vi "Programacion paralela.vi"() -> ()   [LabVIEW 2020]
panel:
  out "Thermometer 6":u16(slide) scale=0.0..100.0
  out "Thermometer 5":u16(slide) scale=0.0..100.0
  out "Thermometer 4":u16(slide) scale=0.0..100.0
  out "Thermometer 3":u16(slide) scale=0.0..100.0
  out "Thermometer 2":u16(slide) scale=0.0..100.0
  out "Thermometer":u16(slide) scale=0.0..100.0
  # "´Programacion PARALELA"
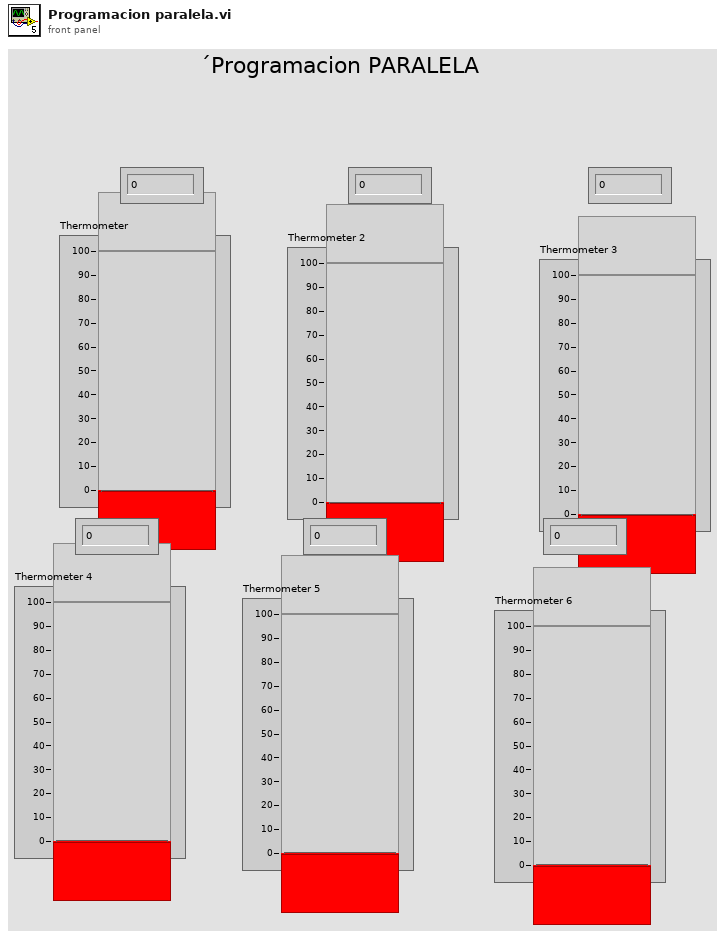
[diagram p1: front panel]
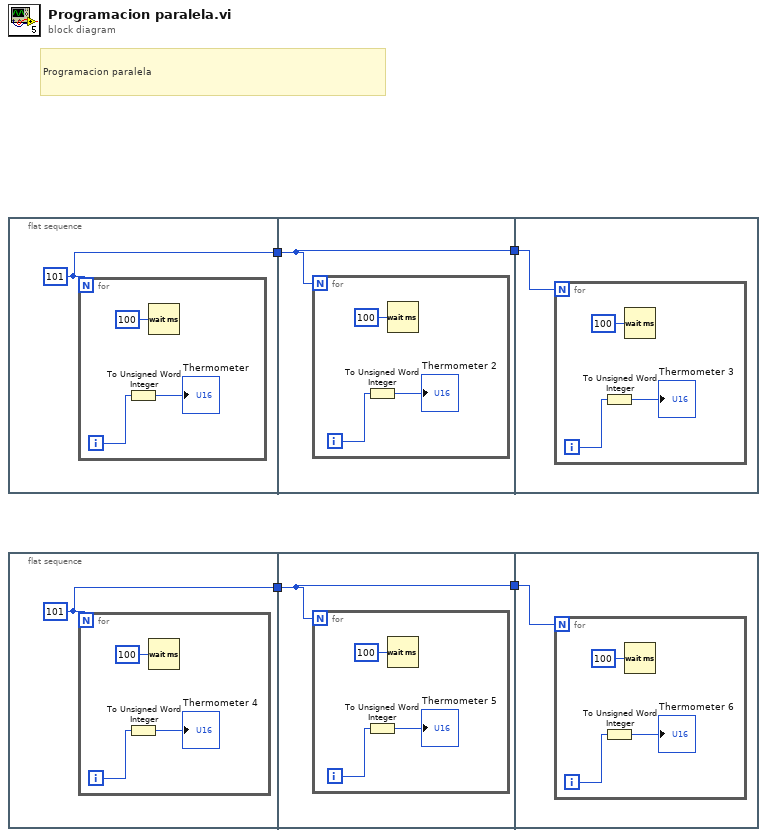
[diagram p0: block diagram]
diagram:
  # "Programacion paralela"
  n1 = flat-sequence {
    tunnel: [w5] -> w4
    tunnel: w4 -> [w9]
    tunnel: [w9] -> w3
    tunnel: w3 -> [w13]
    frame #0 {
      w5 = 101
      n2 = for {
        N: w5 -> [_]
        i -> [w7]
        n3 = To Unsigned Word Integer(number=w7) -> (unsigned 16bit integer=→"Thermometer":u16)
        n4 = Wait (ms)(milliseconds to wait=u32 100) -> ()  [unwired: 1 out]
      }
    }
    frame #1 {
      n5 = for {
        N: w9 -> [_]
        i -> [w11]
        n6 = To Unsigned Word Integer(number=w11) -> (unsigned 16bit integer=→"Thermometer 2":u16)
        n7 = Wait (ms)(milliseconds to wait=u32 100) -> ()  [unwired: 1 out]
      }
    }
    frame #2 {
      n8 = for {
        N: w13 -> [_]
        i -> [w15]
        n9 = To Unsigned Word Integer(number=w15) -> (unsigned 16bit integer=→"Thermometer 3":u16)
        n10 = Wait (ms)(milliseconds to wait=u32 100) -> ()  [unwired: 1 out]
      }
    }
  }
  n11 = flat-sequence {
    tunnel: [w17] -> w2
    tunnel: w2 -> [w21]
    tunnel: [w21] -> w1
    tunnel: w1 -> [w25]
    frame #0 {
      w17 = 101
      n12 = for {
        N: w17 -> [_]
        i -> [w19]
        n13 = To Unsigned Word Integer(number=w19) -> (unsigned 16bit integer=→"Thermometer 4":u16)
        n14 = Wait (ms)(milliseconds to wait=u32 100) -> ()  [unwired: 1 out]
      }
    }
    frame #1 {
      n15 = for {
        N: w21 -> [_]
        i -> [w23]
        n16 = To Unsigned Word Integer(number=w23) -> (unsigned 16bit integer=→"Thermometer 5":u16)
        n17 = Wait (ms)(milliseconds to wait=u32 100) -> ()  [unwired: 1 out]
      }
    }
    frame #2 {
      n18 = for {
        N: w25 -> [_]
        i -> [w27]
        n19 = To Unsigned Word Integer(number=w27) -> (unsigned 16bit integer=→"Thermometer 6":u16)
        n20 = Wait (ms)(milliseconds to wait=u32 100) -> ()  [unwired: 1 out]
      }
    }
  }
